vi "generate default PID.vi"(8 "error in":errorcluster, 11 "PID array in":T2) -> (0 "error out":errorcluster, 2 "PID Array Element":T1={"Loop ID"="", "Tags"={"Setpoint"="", "Process Variable"="", "Output"=""}, "Gains"={"P"=1.0, "I"=0.01, "D"=0.0}, "Range"={"High"=100.0, "Low"=-100.0}})   [LabVIEW 2014, in "Tagbus PID Module editor node.lvclass"]
uses:
  Tagbus PID Module editor node.lvclass
  PID array reference.ctl
  PID array element.ctl
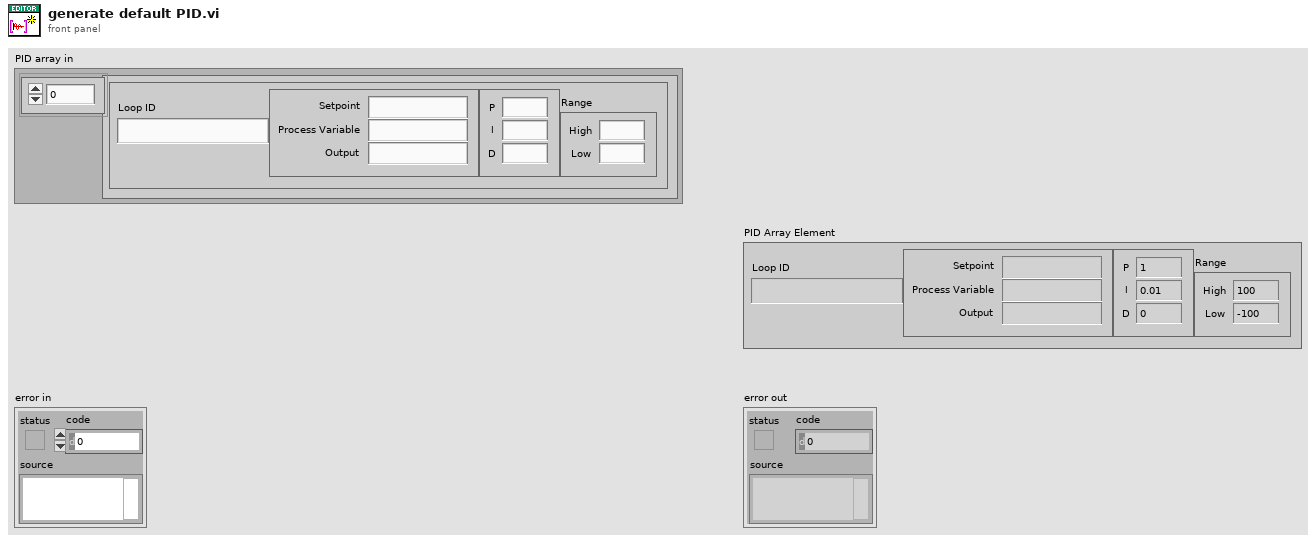
[diagram p1: front panel]
types:
  T1 = typedef "Tagbus PID Module editor node.lvclass/PID array element.ctl" = cluster{"Loop ID":string, "Tags":cluster{"Setpoint":string, "Process Variable":string, "Output":string}, "Gains":cluster{"P":dbl, "I":dbl, "D":dbl}, "Range":cluster{"High":dbl, "Low":dbl}}
  T2 = typedef "Tagbus PID Module editor node.lvclass/PID array reference.ctl" = refnum<vi>
  T3 = cluster{"proportional gain (Kc)":dbl, "integral time (Ti, min)":dbl, "derivative time (Td, min)":dbl}
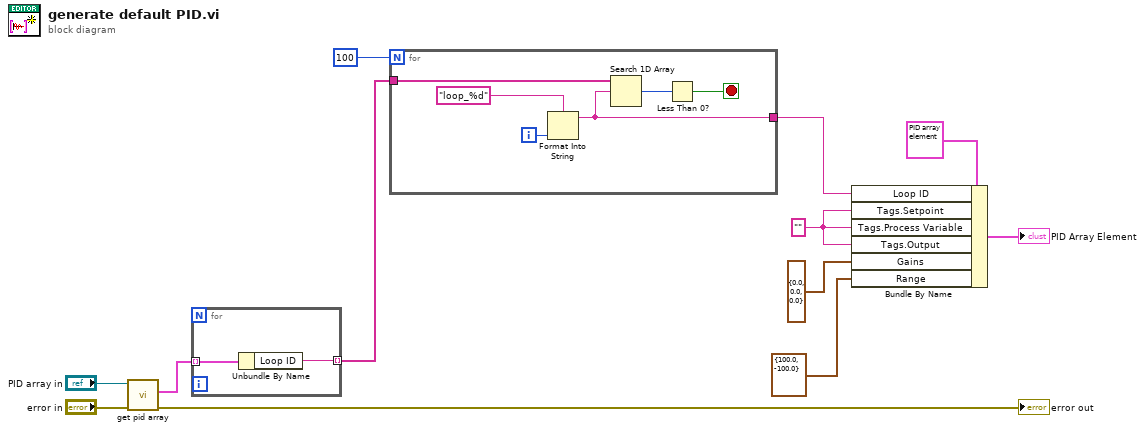
[diagram p0: block diagram]
diagram:
  w5 = "" ("Tags.Setpoint")
  n1 = call "get pid array.vi"("error in (no error)"="error in", "Array in"="PID array in") -> ("error out"=→"error out":errorcluster, "Value"=w2:T1[])  [unwired: 7 in, 1 out]
  n2 = for {
    tunnel: [w14] -> w11 mode=indexing
    tunnel: w2 -> [w13] mode=indexing
    n3 = Unbundle By Name(w13) -> ("Loop ID"=w14:string)
  }
  n4 = for {
    N: 100 -> [_]
    tunnel: w11 -> [w18]
    tunnel: [w15] -> w6
    i -> [w20]
    stop <- w16 stop-if-true
    n5 = Format Into String(format string="loop_%d", w20) -> (resulting string=w15:string)  [unwired: 2 in, 1 out]
    n6 = Search 1D Array(1D array=w18, element=w15) -> (index of element=w17:i32)  [unwired: 1 in]
    n7 = Less Than 0?(x=w17) -> (x < 0?=w16:bool)
  }
  n8 = Bundle By Name(cluster=T1 {"Loop ID"="", "Tags"={"Setpoint"="", "Process Variable"="", "Output"=""}, "Gains"={"P"=1.0, "I"=0.01, "D"=0.0}, "Range"={"High"=100.0, "Low"=-100.0}} ("line"), "Loop ID"=w6, "Tags.Setpoint"=w5, "Tags.Process Variable"=w5, "Tags.Output"=w5, "Gains"=T3 {"proportional gain (Kc)"=0.0, "integral time (Ti, min)"=0.0, "derivative time (Td, min)"=0.0} ("PID gains"), "Range"=cluster{"output high":dbl, "output low":dbl} {"output high"=100.0, "output low"=-100.0} ("output range")) -> (→"PID Array Element":T1)
